vi "_nimcDMControlLoop_Add(32.16).vi"(2 "Fraction B":i16, 3 "Integer B":i32, 4 "Fraction A":i16, 5 "Integer A":i32) -> (0 "Fraction C":i16, 1 "Integer C":i32)   [LabVIEW 2014]
doc: "Performs fixed point addition with 32.16 operands and result."
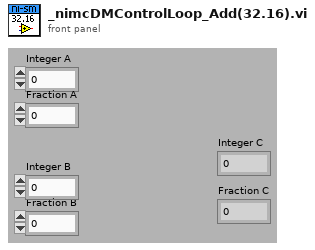
[diagram p1: front panel]
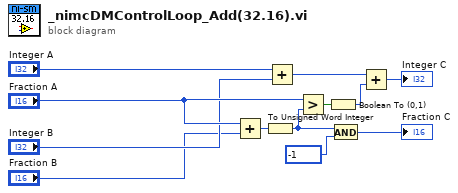
[diagram p0: block diagram]
diagram:
  n1 = Add(x="Fraction A", y="Fraction B") -> (x+y=w9:i16)
  n2 = To Unsigned Word Integer(number=w9) -> (unsigned 16bit integer=w1:u16)
  n3 = Add(x="Integer A", y="Integer B") -> (x+y=w10:i32)
  n4 = Greater?(x="Fraction A", y=w1) -> (0:w12:bool)
  n5 = Boolean To (0,1)(Boolean=w12) -> (0, 1=w11:i16)
  n6 = And(x=w1, y=i16 -1) -> (x .and. y?=→"Fraction C":u16)
  n7 = Add(x=w10, y=w11) -> (x+y=→"Integer C":i32)
